vi "GetAttributeViReal64.vi"(8 "error in (no error)":errorcluster {"code" format="%.0x"}, 9 "AttributeID":u32(ring)=1150011 items=["ROUTE_MONITOR_DATA"=1150011, "ROUTE_MONITOR_FULL_DATA"=1150069, "SCAN_SINGLE_CHANNEL_SAMPLE_INTERVAL"=1150064, "SCAN_TIMER_INTERVAL"=1150029, "SCAN_TRIGGER_DELAY"=1150059, "SCAN_TRIGGER_LEVEL"=1150060, "SYSTEM_LINE_FREQUENCY"=1150037], 11 "instrument handle":refnum<k15>) -> (0 "error out":errorcluster {"code" format="%.0x"}, 2 "AttributeValue":dbl, 3 "instrument handle out":refnum<k15>)   [LabVIEW 2020, in "Keysight DAQ970.lvlib"]
doc: "Gets a Real64 attribute from the instrument driver.\nThe following Attributes are supported:\n\nROUTE_MONITOR_DATA\n\nROUTE_MONITOR_FULL_DATA \n\nSCAN_SINGLE_CHANNEL_SAMPLE_INTERVAL\n\nSCAN_TIMER_INTERVAL\n\nSCAN_TRIGGER_DELAY\n\nSCAN_TRIGGER_LEVEL\n\nSYSTEM_LINE_FREQUENCY"
uses:
  Keysight DAQ970.lvlib
  KtDAQ970.dll
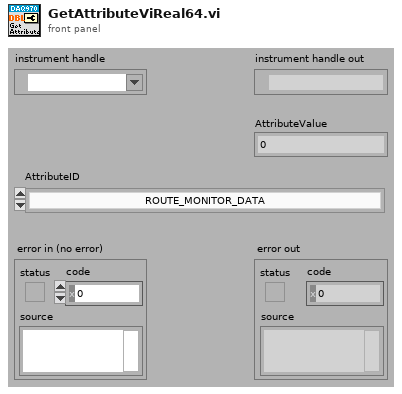
[diagram p1: front panel]
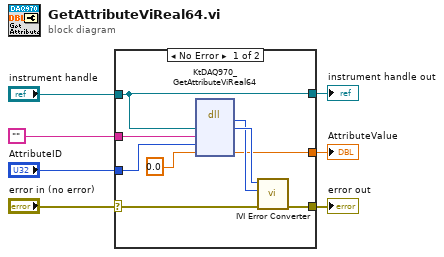
[diagram p0: block diagram]
diagram:
  n1 = case shown="No Error" "error in (no error)" {
    selector: "error in (no error)" -> [w14 w18]
    tunnel: [w13 w18] -> w7
    tunnel: "instrument handle" -> [w8 w17]
    tunnel: "" -> [w12 _]
    tunnel: "AttributeID" -> [w11 _]
    tunnel: [w9 _] -> w4
    tunnel: [w8 w17] -> w2
    frame No Error {
      n2 = dll-call lib="KtDAQ970**.dll" fn="KtDAQ970_GetAttributeViReal64"("Vi"=w8, "RepCapIdentifier"=w12, "AttributeID"=w11, "AttributeValue"=0.0) -> ("return type"=w15:i32, "Vi"=w16:u32, "AttributeValue"=w9:dbl)  [unwired: 5 in, 2 out]
      n3 = call "IVI Error Converter.vi"("error in (no error)"=w14, "IVI error code (0)"=w15, "instrument handle"=w16) -> ("error out"=w13:errorcluster)  [unwired: 7 in, 1 out]
    }
    frame Error {
    }
  }
  "error out" <- w7
  "instrument handle out" <- w2
  "AttributeValue" <- w4
